vi "Config Low Frequency Output.vi"(0 "VISA Resource Name":refnum<visa-resource-name>, 1 "LF Out Source (0:Internal)":enum16{"INTERNAL", "FUNCTION GENERATOR"}(ring), 2 "Frequency (400.0)":dbl=400.0 format="%.1f", 3 "LF Out Waveform (0:SINE)":T2(ring), 5 "LF Out (T:ON)":bool=TRUE, 7 "LF Out Amplitude (0)":dbl format="%.3f", 11 "error in (no error)":errorcluster {"code" format="%.0x"}, 12 "Dual/Swept/Pulse Parameters":T1={"Alt Frequency (400.0)"=400.0, "Alt Freq Amplitude (50.0)"=50.0, "Sweep Time (100.0)"=100.0, "Sweep Trigger (0:IMMEDIATE)"=enum."IMMEDIATE", "Pulse Period (80.0)"=80.0, "Pulse Width (40.0)"=40.0} {"Pulse Width (40.0)" format="%.1f"; "Pulse Period (80.0)" format="%.1f"; "Sweep Time (100.0)" format="%.1f"; "Alt Freq Amplitude (50.0)" format="%.1f"; "Alt Frequency (400.0)" format="%.1f"}) -> (4 "VISA Resource Name Out":refnum<visa-resource-name>, 15 "error out":errorcluster {"code" format="%.0x"})   [LabVIEW 2012, in "Agilent ESG Series.lvlib"]
doc: "This VI is used to set the controls and the parameters associated with the low frequency output signals."
uses:
  <instrlib>/Agilent ESG Series/Agilent ESG Series.lvlib
panel:
  # "ON"
  # "OFF"
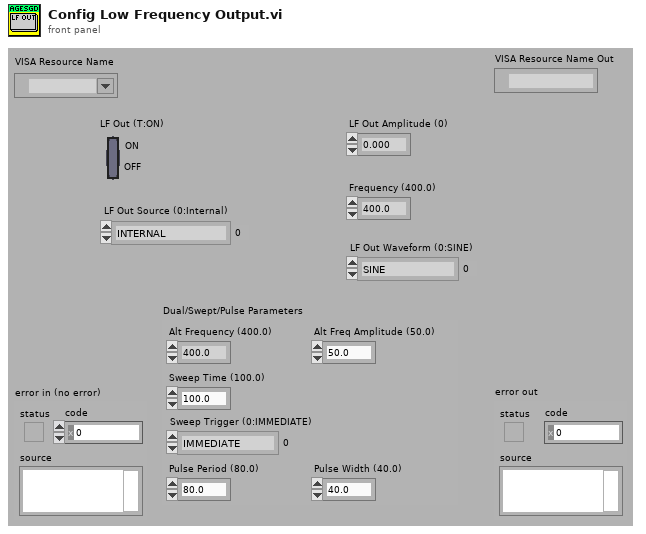
[diagram p1: front panel]
types:
  T1 = cluster{"Alt Frequency (400.0)":dbl, "Alt Freq Amplitude (50.0)":dbl, "Sweep Time (100.0)":dbl, "Sweep Trigger (0:IMMEDIATE)":enum16{"IMMEDIATE", "BUS", "EXTERNAL", "KEY"}, "Pulse Period (80.0)":dbl, "Pulse Width (40.0)":dbl}
  T2 = enum16{"SINE", "TRIANGLE", "SQUARE", "RAMP", "NOISE", "DC", "DUAL SINE", "SWEPT SINE", "PULSE"}
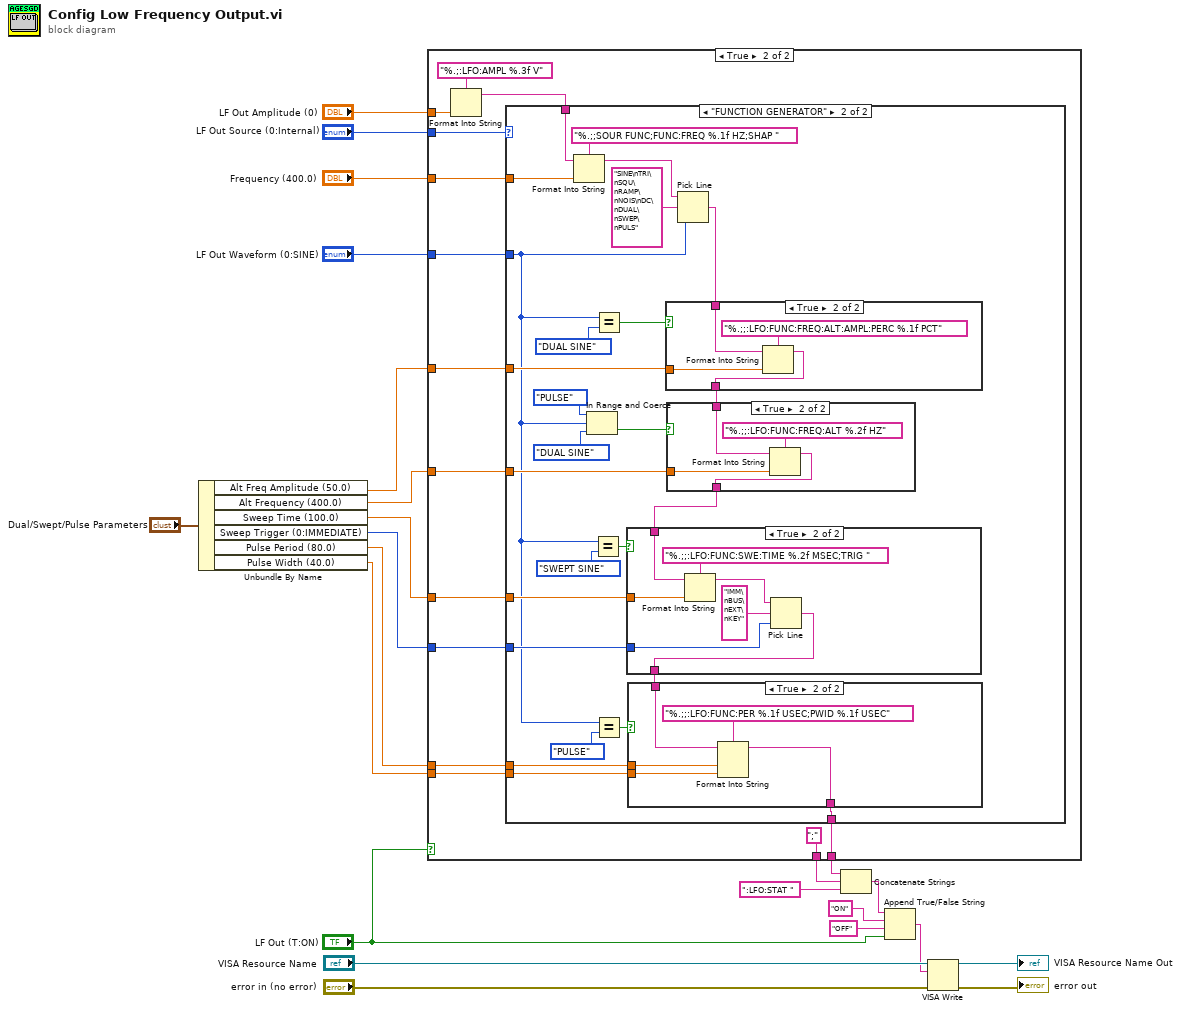
[diagram p0: block diagram]
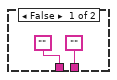
[diagram p2: hidden frame]
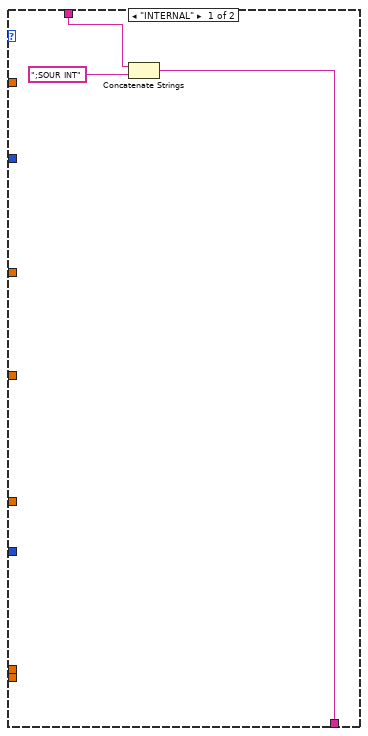
[diagram p3: hidden frame]
diagram:
  n1 = Unbundle By Name("Dual/Swept/Pulse Parameters") -> ("Alt Freq Amplitude (50.0)"=w6:dbl, "Alt Frequency (400.0)"=w5:dbl, "Sweep Time (100.0)"=w4:dbl, "Sweep Trigger (0:IMMEDIATE)"=w3:enum16{"IMMEDIATE", "BUS", "EXTERNAL", "KEY"}, "Pulse Period (80.0)"=w2:dbl, "Pulse Width (40.0)"=w1:dbl)
  n2 = case shown="True" "LF Out (T:ON)" {
    tunnel: ["" w39] -> w10
    tunnel: w1 -> [_ w38]
    tunnel: w2 -> [_ w37]
    tunnel: w3 -> [_ w36]
    tunnel: w4 -> [_ w35]
    tunnel: w6 -> [_ w34]
    tunnel: w5 -> [_ w33]
    tunnel: "LF Out Waveform (0:SINE)" -> [_ w32]
    tunnel: "Frequency (400.0)" -> [_ w30]
    tunnel: "LF Out Source (0:Internal)" -> [_ w29]
    tunnel: "LF Out Amplitude (0)" -> [_ w28]
    tunnel: ["" ";"] -> w9
    frame False {
    }
    frame True {
      n3 = Format Into String(format string="%.;:LFO:AMPL %.3f V", w28) -> (resulting string=w31:string)  [unwired: 2 in, 1 out]
      n4 = case shown="\"FUNCTION GENERATOR\"" w29 {
        tunnel: w31 -> [w42 w68]
        tunnel: [w40 w52] -> w39
        tunnel: w30 -> [_ w67]
        tunnel: w32 -> [_ w43]
        tunnel: w33 -> [_ w46]
        tunnel: w34 -> [_ w63]
        tunnel: w36 -> [_ w58]
        tunnel: w35 -> [_ w59]
        tunnel: w37 -> [_ w54]
        tunnel: w38 -> [_ w53]
        frame "INTERNAL" {
          n5 = Concatenate Strings(w42, ";SOUR INT") -> (w40:string)
        }
        frame "FUNCTION GENERATOR" {
          n6 = Format Into String(format string="%.;;SOUR FUNC;FUNC:FREQ %.1f HZ;SHAP ", initial string=w68, w67) -> (resulting string=w64:string)  [unwired: 1 in, 1 out]
          n7 = In Range and Coerce(upper limit=T2."PULSE" ("hi"), x=w43, lower limit=T2."DUAL SINE" ("y")) -> (In Range?=w51:bool)  [unwired: 1 out]
          n8 = Equal?(x=w43, y=T2."SWEPT SINE") -> (x = y?=w61:bool)
          n9 = Equal?(x=w43, y=T2."DUAL SINE" ("hi")) -> (x = y?=w49:bool)
          n10 = Equal?(x=w43, y=T2."PULSE") -> (x = y?=w56:bool)
          n11 = Pick Line(string ("")=w64, multi-line string="SINE\nTRI\nSQU\nRAMP\nNOIS\nDC\nDUAL\nSWEP\nPULS", line index=w43) -> (output string=w47:string)
          n12 = case shown="True" w49 {
            tunnel: [w69 w72] -> w50
            tunnel: w47 -> [w69 w70]
            tunnel: w63 -> [_ w71]
            frame False {
            }
            frame True {
              n13 = Format Into String(format string="%.;;:LFO:FUNC:FREQ:ALT:AMPL:PERC %.1f PCT", initial string=w70, w71) -> (resulting string=w72:string)  [unwired: 1 in, 1 out]
            }
          }
          n14 = case shown="True" w51 {
            tunnel: w50 -> [w74 w75]
            tunnel: [w74 w77] -> w60
            tunnel: w46 -> [_ w76]
            frame False {
            }
            frame True {
              n15 = Format Into String(format string="%.;;:LFO:FUNC:FREQ:ALT %.2f HZ", initial string=w75, w76) -> (resulting string=w77:string)  [unwired: 1 in, 1 out]
            }
          }
          n16 = case shown="True" w61 {
            tunnel: w60 -> [w85 w86]
            tunnel: [w85 w89] -> w55
            tunnel: w59 -> [_ w88]
            tunnel: w58 -> [_ w87]
            frame False {
            }
            frame True {
              n17 = Format Into String(format string="%.;;:LFO:FUNC:SWE:TIME %.2f MSEC;TRIG ", initial string=w86, w88) -> (resulting string=w92:string)  [unwired: 1 in, 1 out]
              n18 = Pick Line(string ("")=w92, multi-line string="IMM\nBUS\nEXT\nKEY", line index=w87) -> (output string=w89:string)
            }
          }
          n19 = case shown="True" w56 {
            tunnel: w55 -> [w79 w82]
            tunnel: [w79 w81] -> w52
            tunnel: w54 -> [_ w84]
            tunnel: w53 -> [_ w83]
            frame False {
            }
            frame True {
              n20 = Format Into String(format string="%.;;:LFO:FUNC:PER %.1f USEC;PWID %.1f USEC", initial string=w82, w84, w83) -> (resulting string=w81:string)  [unwired: 1 in, 1 out]
            }
          }
        }
      }
    }
  }
  n21 = Concatenate Strings(w10, w9, ":LFO:STAT ") -> (w18:string)
  n22 = Append True/False String(1:"LF Out (T:ON)", 2:"OFF" ("false string"), 3:"ON" ("true string"), 4:w18) -> (0:w8:string)
  n23 = VISA Write(VISA resource name="VISA Resource Name", write buffer=w8, error in (no error)="error in (no error)") -> (VISA resource name out=→"VISA Resource Name Out":refnum<visa-resource-name>, error out=→"error out":errorcluster)  [unwired: 1 out]
